vi "GetLibraryDependencies.vi"(11 "FileDependency":map{path, T1}(c390)) -> (2 "LibraryDependency":map{path, T3}(c390))   [LabVIEW 2020, in "DependencyChecker.lvlib"]
uses:
  DependencyChecker.lvlib
  LibraryDependentInfo.vi
  <vilib>/Utility/lvfile.llb/FT_FileTypes.ctl
  FileDependencyType.ctl
  <vilib>/Utility/miscctls.llb/LVMapReplaceAction.ctl
  <vilib>/Utility/lvfile.llb/NI_FileType.lvlib
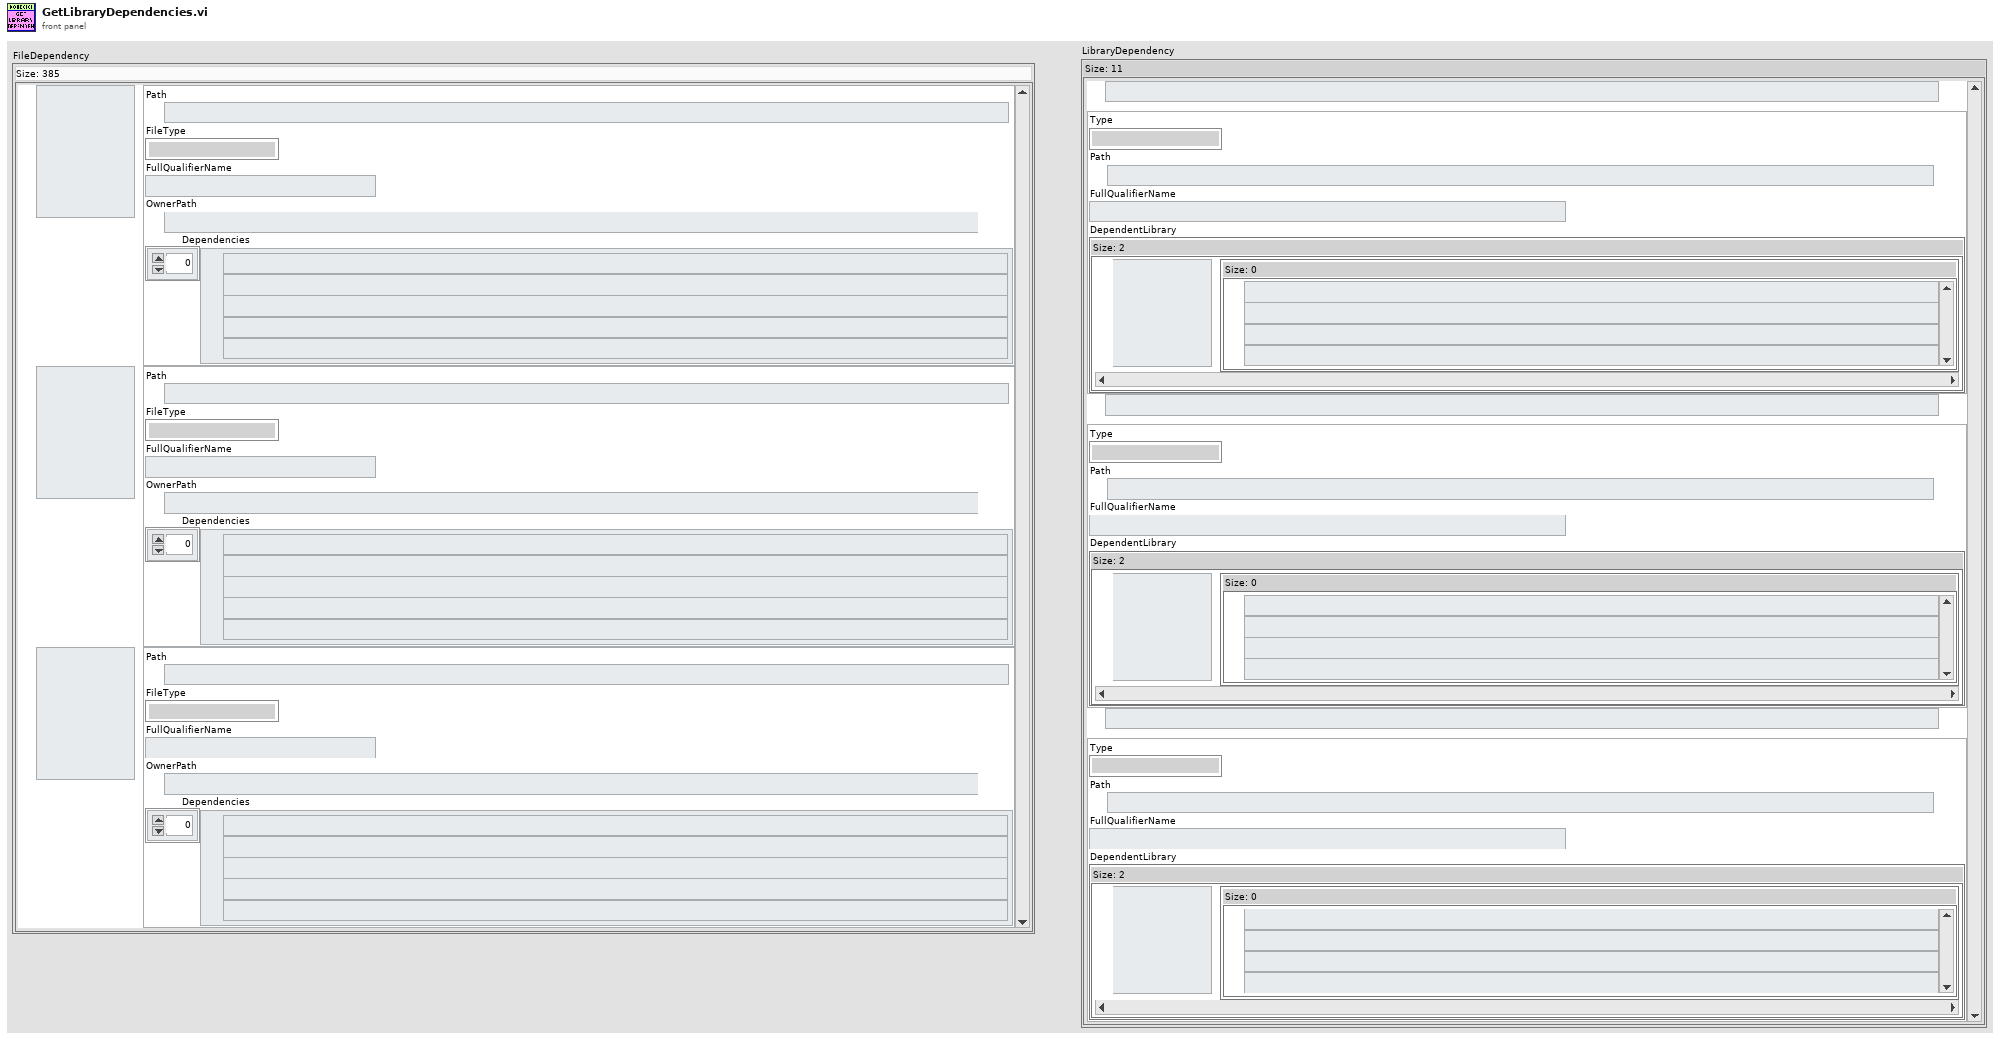
[diagram p1: front panel]
types:
  T1 = typedef "DependencyChecker.lvlib/FileDependencyType.ctl" = cluster{"Path":path, "FileType":T2, "FullQualifierName":string, "OwnerPath":path, "Dependencies":path[]}
  T2 = typedef "NI_FileType.lvlib/FT_FileTypes.ctl" = enum32{"Invalid file/path", "Unknown type", "Instrument", "Control", "Polymorphic VI", "Project", "Library", "LVClass", "XControl", "XNode", "CIN", "Run-time menu", "Palette menu", "LLB", "Shortcut", "Directory", "Class Private Data Control", "Statechart", "MathScript .m file", "Ladder Diagram", "LVLibp"}
  T3 = typedef "DependencyChecker.lvlib/LibraryDependentInfo.vi" = cluster{"Type":T2, "Path":path, "FullQualifierName":string, "DependentLibrary":map{path, set{path}}}
  T4 = typedef "LVMapReplaceAction.ctl" = enum32{"Modify Entry only if found", "Add or Modify Entry", "Delete Entry"}
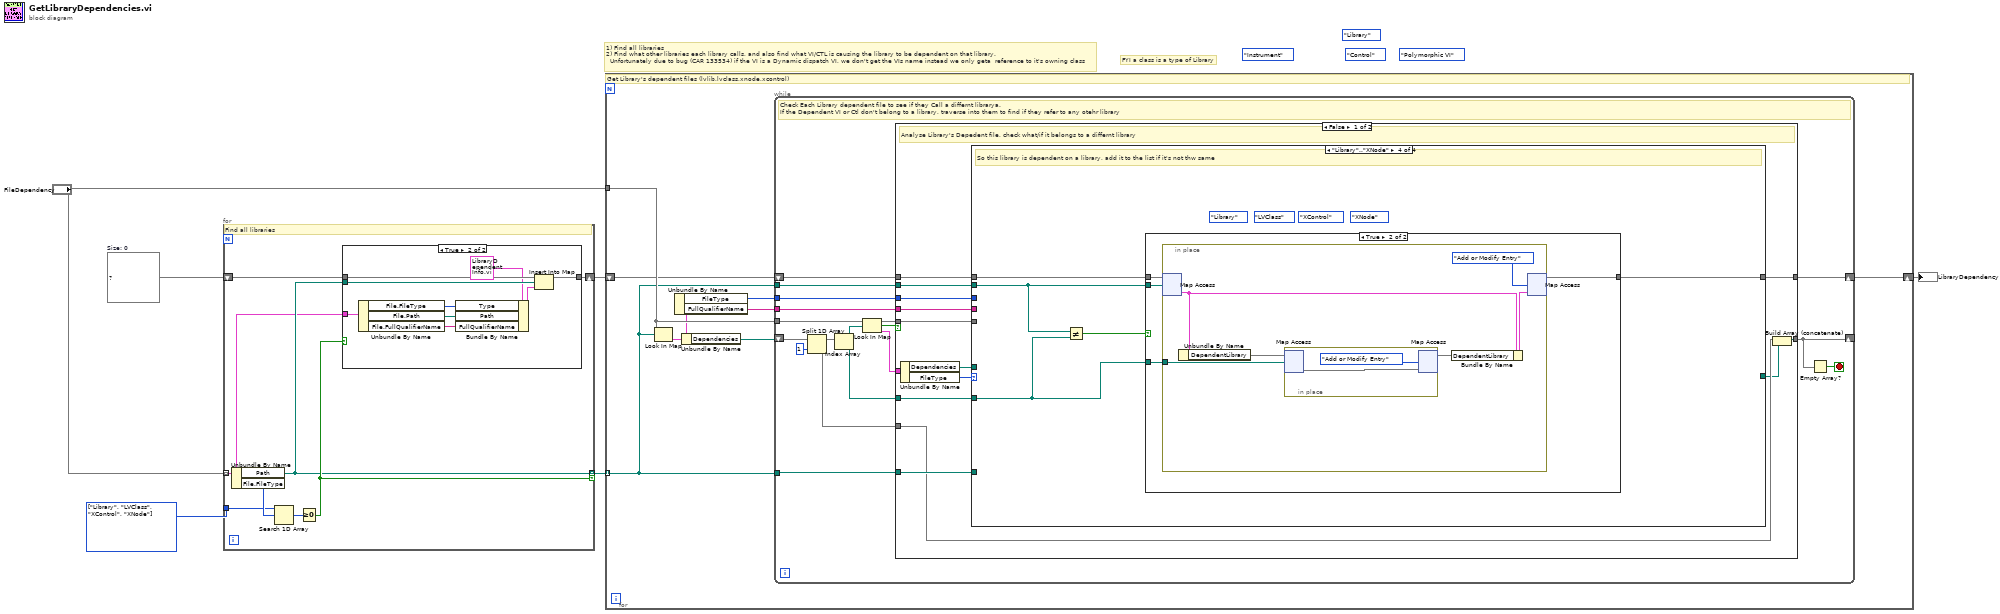
[diagram p0: block diagram]
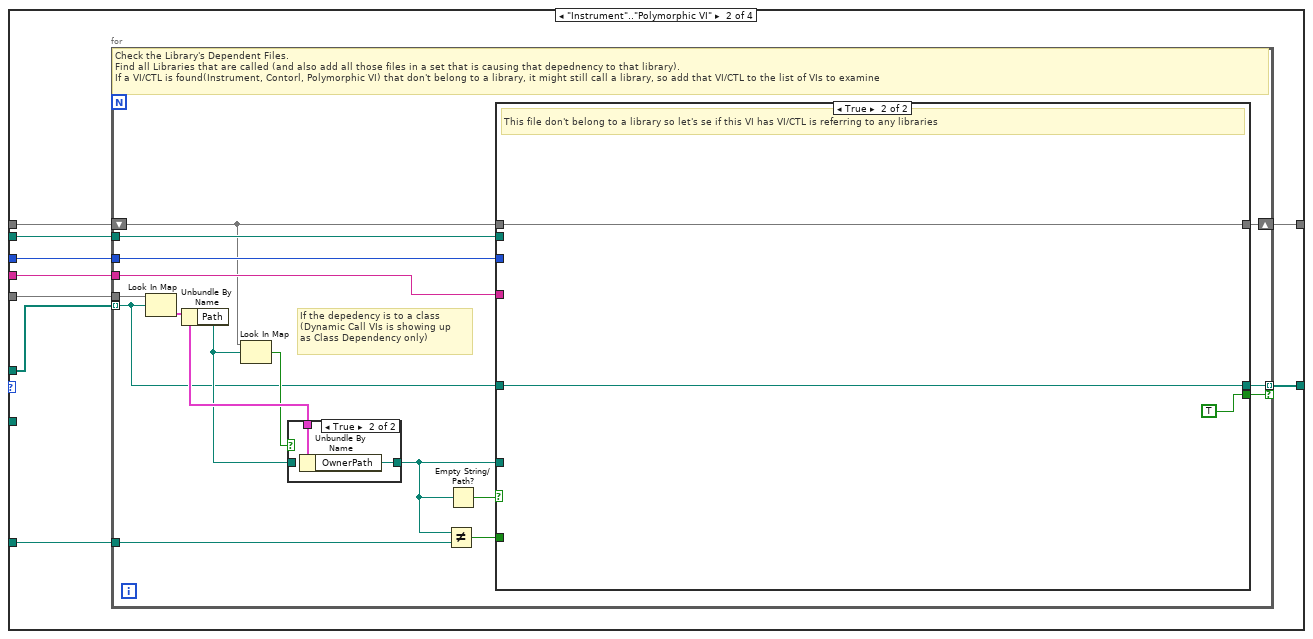
[diagram p3: hidden frame]
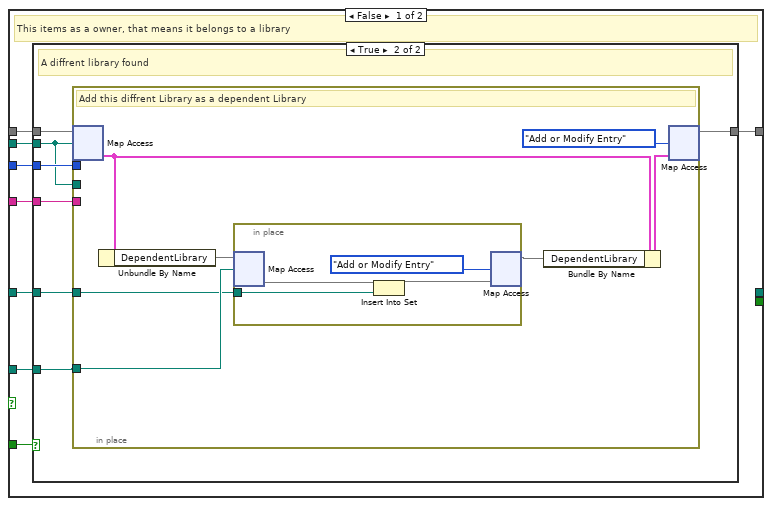
[diagram p4: hidden frame]
diagram:
  (unwired) FT_FileTypes."Library" ("FileType")
  (unwired) FT_FileTypes."Instrument" ("FileType")
  (unwired) FT_FileTypes."Control" ("FileType")
  (unwired) FT_FileTypes."Polymorphic VI" ("FileType")
  w5 = map{path, T3} {}  # Size: 0
  w3 = T2[] [enum."Library", enum."LVClass", enum."XControl", enum."XNode"] items=["Invalid file/path", "Unknown type", "Instrument", "Control", "Polymorphic VI", "Project", "Library", "LVClass", "XControl", "XNode", "CIN", "Run-time menu", "Palette menu", "LLB", "Shortcut", "Directory", "Class Private Data Control", "Statechart", "MathScript .m file", "Ladder Diagram", "LVLibp"] ("y")
  # "1) Find all libraries \n2) Find what other libraries each library calls, and also find what VI/CTL is causing the library to be dependent on that library.\n  Unfortunately due to bug (CAR 133534) if the VI is a Dynamic dispatch VI, we don't get the VIs name instead we only geta  reference to it's owning class"
  # "FYI a class is a type of Library"
  n1 = for {
    tunnel: "FileDependency" -> [w7] mode=indexing
    tunnel: [w8] -> w1 mode=indexing if=w11
    tunnel: w3 -> [w12]
    shift-right: [w9] -> w6
    shift-left: w5 -> [w10]
    # "Find all libraries"
    n2 = Unbundle By Name(w7) -> ("Path"=w8:path, "File.FileType"=w13:T2)
    n3 = Search 1D Array(1D array=w12, element=w13) -> (index of element=w14:i32)  [unwired: 1 in]
    n4 = Greater Or Equal To 0?(x=w14) -> (x >= 0?=w11:bool)
    n5 = case shown="True" w11 {
      tunnel: w10 -> [w15 w24]
      tunnel: [w15 w23] -> w9
      tunnel: w8 -> [_ w22]
      tunnel: w7 -> [_ w19]
      frame False {
      }
      frame True {
        n6 = Unbundle By Name(w19) -> ("File.FileType"=w18:T2, "File.Path"=w17:path, "File.FullQualifierName"=w16:string)
        n7 = Bundle By Name(cluster=T3 {"Type"=enum."Library", "Path"=path "", "FullQualifierName"="", "DependentLibrary"={}} ("LibraryDependentInfo"), "Type"=w18, "Path"=w17, "FullQualifierName"=w16) -> (w20:T3)
        n8 = Insert Into Map(map in=w24, key=w22, value=w20) -> (map out=w23:map{path, T3})  [unwired: 2 out]
      }
    }
  }
  n9 = for {
    tunnel: w1 -> [w25] mode=indexing
    tunnel: "FileDependency" -> [w31]
    shift-right: [w29] -> w4
    shift-left: w6 -> [w30]
    # "Get Library's dependent files (lvlib,lvclass,xnode,xcontrol)"
    n10 = Look In Map(map=w31, key=w25) -> (value=w28:T1)  [unwired: 1 in, 1 out]
    n11 = Unbundle By Name(w28) -> ("FileType"=w27:T2, "FullQualifierName"=w26:string)
    n12 = Unbundle By Name(w28) -> ("Dependencies"=w32:path[])
    n13 = while {
      tunnel: w31 -> [w47]
      tunnel: w25 -> [w46]
      shift-right: [w44] -> w29
      shift-left: w30 -> [w45]
      tunnel: w27 -> [w43]
      tunnel: w26 -> [w42]
      tunnel: w25 -> [w41]
      shift-right: [w37] -> _
      shift-left: w32 -> [w38]
      stop <- w36 stop-if-true
      # "Check Each Library dependent file to see if they Call a differnt librarya.\nIf the Dependent VI or Ctl don't belong to a library, traverse into them to find if they refer to any otehr library"
      n14 = Split 1D Array(array=w38, index=1) -> (first subarray=w39:path[], second subarray=w33:path[])
      n15 = Index Array(array=w39) -> (element=w34:path)  [unwired: 1 in]
      n16 = Look In Map(map=w47, key=w34) -> (key not found?=w35:bool, value=w48:T1)  [unwired: 1 in]
      n17 = case shown="False" w35 {
        tunnel: w48 -> [w62 _]
        tunnel: w47 -> [w61 _]
        tunnel: w46 -> [w59 _]
        tunnel: w45 -> [w58 w142]
        tunnel: [w57 w142] -> w44
        tunnel: w43 -> [w56 _]
        tunnel: w42 -> [w55 _]
        tunnel: w41 -> [w54 _]
        tunnel: w34 -> [w52 _]
        tunnel: [w50 w141] -> w37
        tunnel: w33 -> [w51 w141]
        frame False {
          # "Analyse Library's Depedent file, check what/if it belongs to a differnt library"
          n18 = Unbundle By Name(w62) -> ("Dependencies"=w60:path[], "FileType"=w53:T2)
          n19 = case shown="\"Library\"..\"XNode\"" w53 {
            tunnel: w61 -> [_ w72 _ _]
            tunnel: w60 -> [_ w71 _ _]
            tunnel: w59 -> [_ w70 _ _]
            tunnel: w58 -> [w63 w69 w122 w127]
            tunnel: [w63 w68 w122 w126] -> w57
            tunnel: w56 -> [_ w67 _ _]
            tunnel: w55 -> [_ w66 _ _]
            tunnel: w54 -> [_ w65 _ w124]
            tunnel: w52 -> [_ _ _ w125]
            tunnel: [_ w64 _ _] -> w49
            frame "Class Private Data Control" {
            }
            frame "Instrument".."Polymorphic VI" {
              n20 = for {
                tunnel: w72 -> [w88]
                tunnel: w71 -> [w77] mode=indexing
                tunnel: w70 -> [w87]
                shift-right: [w86] -> w68
                shift-left: w69 -> [w81]
                tunnel: w65 -> [w85]
                tunnel: w67 -> [w84]
                tunnel: w66 -> [w83]
                tunnel: [w74] -> w64 mode=indexing if=w73
                # "If the depedency is to a class\n(Dynamic Call VIs is showing up \nas Class Dependency only)"
                # "Check the Library's Dependent Files.\nFind all Libraries that are called (and also add all those files in a set that is causing that depednency to that library).\nIf a VI/CTL is found(Instrument, Contorl, Polymorphic VI) that don't belong to a library, it might still call a library, so add that VI/CTL to the list of VIs to examine"
                n21 = Look In Map(map=w88, key=w77) -> (value=w80:T1)  [unwired: 1 in, 1 out]
                n22 = Unbundle By Name(w80) -> ("Path"=w78:path)
                n23 = Look In Map(map=w81, key=w78) -> (key not found?=w79:bool)  [unwired: 1 in, 1 out]
                n24 = case shown="True" w79 {
                  tunnel: [w119 w121] -> w82
                  tunnel: w80 -> [_ w120]
                  tunnel: w78 -> [w119 _]
                  frame False {
                  }
                  frame True {
                    n25 = Unbundle By Name(w120) -> ("OwnerPath"=w121:path)
                  }
                }
                n26 = Not Equal?(x=w82, y=w87) -> (x != y?=w76:bool)
                n27 = Empty String/Path?(string/path=w82) -> (empty?=w75:bool)
                n28 = case shown="True" w75 {
                  tunnel: [w96 w118] -> w86
                  tunnel: w85 -> [w95 _]
                  tunnel: w84 -> [w94 _]
                  tunnel: w83 -> [w93 _]
                  tunnel: w82 -> [w92 _]
                  tunnel: w81 -> [w91 w118]
                  tunnel: w77 -> [w90 w117]
                  tunnel: w76 -> [w89 _]
                  tunnel: [_ w117] -> w74
                  tunnel: [_ TRUE] -> w73
                  frame False {
                    # "This items as a owner, that means it belongs to a library"
                    n29 = case shown="True" w89 {
                      tunnel: w91 -> [w97 w104]
                      tunnel: [w97 w98] -> w96
                      tunnel: w95 -> [_ w102]
                      tunnel: w94 -> [_ w103]
                      tunnel: w93 -> [_ w101]
                      tunnel: w92 -> [_ w100]
                      tunnel: w90 -> [_ w99]
                      frame False {
                        # "This VI/CTL belongs to this library, but we want to find other libraries this library is dependent on"
                      }
                      frame True {
                        # "A diffrent library found"
                        n30 = in-place {
                          in-place-border: w103 -> [_]
                          in-place-border: w102 -> [_]
                          in-place-border: w101 -> [_]
                          in-place-border: w100 -> [w106]
                          in-place-border: w99 -> [w105]
                          # "Add this diffrent Library as a dependent Library"
                          n31 = in-place-map #1(w104, w102) -> (w109:T3)  [unwired: 1 in, 1 out]
                          n32 = Unbundle By Name(w109) -> ("DependentLibrary"=w108:map{path, set{path}})
                          n33 = in-place {
                            in-place-border: w105 -> [w112]
                            n34 = in-place-map #2(w108, w106) -> (w114:set{path})  [unwired: 1 in, 1 out]
                            n35 = Insert Into Set(10:w112, 11:w114) -> (3:w113:set{path})  [unwired: 1 out]
                            n36 = in-place-map #2(w113, LVMapReplaceAction."Add or Modify Entry" ("action")) -> (w107:map{path, set{path}})  [unwired: 2 out]
                          }
                          n37 = Bundle By Name(cluster=w109, "DependentLibrary"=w107) -> (w110:T3)
                          n38 = in-place-map #1(w110, LVMapReplaceAction."Add or Modify Entry" ("action")) -> (w98:map{path, T3})  [unwired: 2 out]
                        }
                      }
                    }
                  }
                  frame True {
                    # "This file don't belong to a library so let's se if this VI has VI/CTL is referring to any libraries"
                  }
                }
              }
            }
            frame Default {
            }
            frame "Library".."XNode" {
              (unwired) FT_FileTypes."XNode" ("FileType")
              (unwired) FT_FileTypes."XControl" ("FileType")
              (unwired) FT_FileTypes."LVClass" ("FileType")
              (unwired) FT_FileTypes."Library" ("FileType")
              # "So this library is dependent on a library, add it to the list if it's not thw same"
              n39 = Not Equal?(x=w124, y=w125) -> (x != y?=w123:bool)
              n40 = case shown="True" w123 {
                tunnel: w127 -> [w128 w132]
                tunnel: [w128 w131] -> w126
                tunnel: w125 -> [_ w130]
                tunnel: w124 -> [_ w129]
                frame False {
                }
                frame True {
                  n41 = in-place {
                    in-place-border: w130 -> [w133]
                    n42 = in-place-map #3(w132, w129) -> (w136:T3)  [unwired: 1 in, 1 out]
                    n43 = Unbundle By Name(w136) -> ("DependentLibrary"=w135:map{path, set{path}})
                    n44 = in-place {
                      n45 = in-place-map #4(w135, w133) -> (w139:set{path})  [unwired: 1 in, 1 out]
                      n46 = in-place-map #4(w139, LVMapReplaceAction."Add or Modify Entry" ("action")) -> (w134:map{path, set{path}})  [unwired: 2 out]
                    }
                    n47 = Bundle By Name(cluster=w136, "DependentLibrary"=w134) -> (w137:T3)
                    n48 = in-place-map #3(w137, LVMapReplaceAction."Add or Modify Entry" ("action")) -> (w131:map{path, T3})  [unwired: 2 out]
                  }
                }
              }
            }
          }
          n49 = Build Array (concatenate)(w51, w49) -> (w50:path[])
        }
        frame True {
          # "I guess this VI/CTL don't have any dependency"
        }
      }
      n50 = Empty Array?(array=w37) -> (empty?=w36:bool)
    }
  }
  "LibraryDependency" <- w4
